vi "CameraKill.vi"(8 "error in (no error)":errorcluster, 11 "AndorSDK2 in":refnum<class "Andor2.lvclass">) -> (0 "error out":errorcluster, 3 "AndorSDK2 out":refnum<class "Andor2.lvclass">)   [LabVIEW 2010, in "Andor2.lvclass"]
uses:
  Andor2.lvclass
  Andor2.lvclass/Andor2.ctl
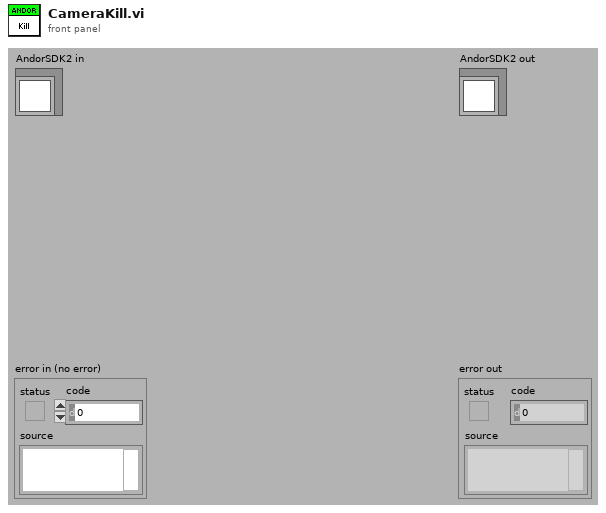
[diagram p1: front panel]
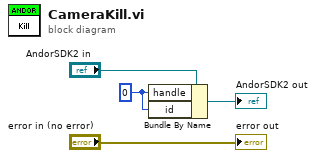
[diagram p0: block diagram]
diagram:
  w3 = 0 ("handle")
  n1 = Bundle By Name(cluster="AndorSDK2 in", "handle"=w3, "id"=w3) -> (→"AndorSDK2 out":refnum<class "Andor2.lvclass">)
  "error out" <- "error in (no error)"
